vi "Read Element of Array.vi"(8 "error in (no error)":errorcluster, 10 "index":i32, 11 "JSON Array in":refnum<class "JSON Array.lvclass">) -> (0 "error out":errorcluster, 2 "JSON Value.lvclass":refnum<class "JSON Value.lvclass">, 3 "JSON Array out":refnum<class "JSON Array.lvclass">)   [LabVIEW 2011, in "JSON Array.lvclass"]
uses:
  JSON Array.lvclass
  JSON Value/JSON Value.lvclass
  JSON Array.lvclass/JSON Array.ctl
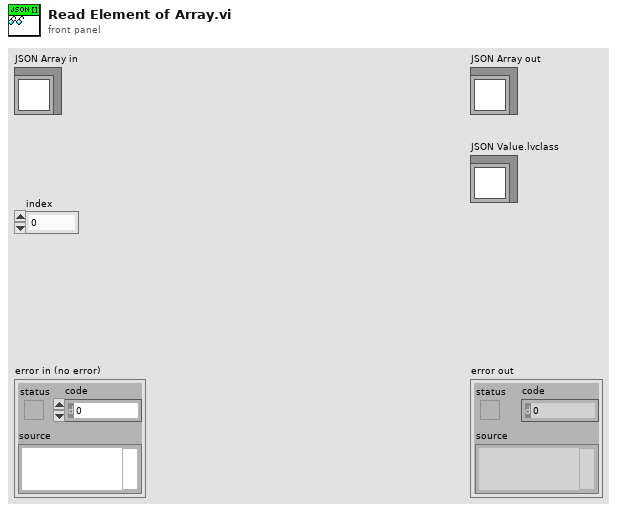
[diagram p1: front panel]
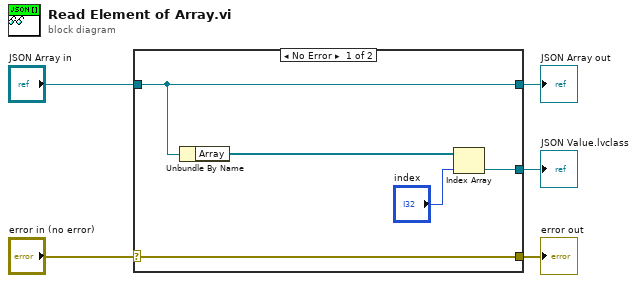
[diagram p0: block diagram]
diagram:
  n1 = case shown="No Error" "error in (no error)" {
    selector: "error in (no error)" -> [w10 w11]
    tunnel: [w10 w11] -> w4
    tunnel: [w9 w12] -> w2
    tunnel: "JSON Array in" -> [w9 w12]
    tunnel: [w6 _] -> w1
    frame No Error {
      n2 = Unbundle By Name(w9) -> ("Array"=w8:refnum<class "JSON Value.lvclass">[])
      n3 = Index Array(array=w8, index="index") -> (element=w6:refnum<class "JSON Value.lvclass">)
    }
    frame Error {
    }
  }
  "error out" <- w4
  "JSON Array out" <- w2
  "JSON Value.lvclass" <- w1
